vi "Read_Array_of_Products_from_File.vi"(11 "Path":path) -> (3 "Array":T1[](array[typedef]))   [LabVIEW 2020]
doc: "This VI reads <b>array of #typedef Products </b> saved in text file stored in location gived by a <b>path</b>. In file every element of cluster is seperated by comma."
uses:
  #typedef_Product.ctl
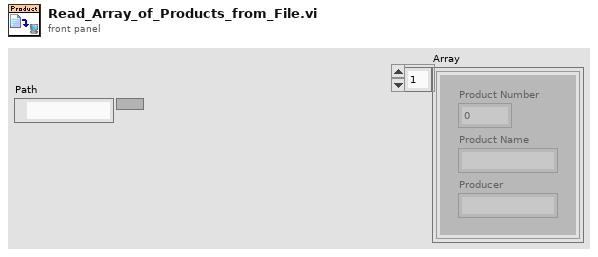
[diagram p1: front panel]
types:
  T1 = typedef "#typedef_Product.ctl" = cluster{"Product Number":i32, "Product Name":string, "Producer":string}
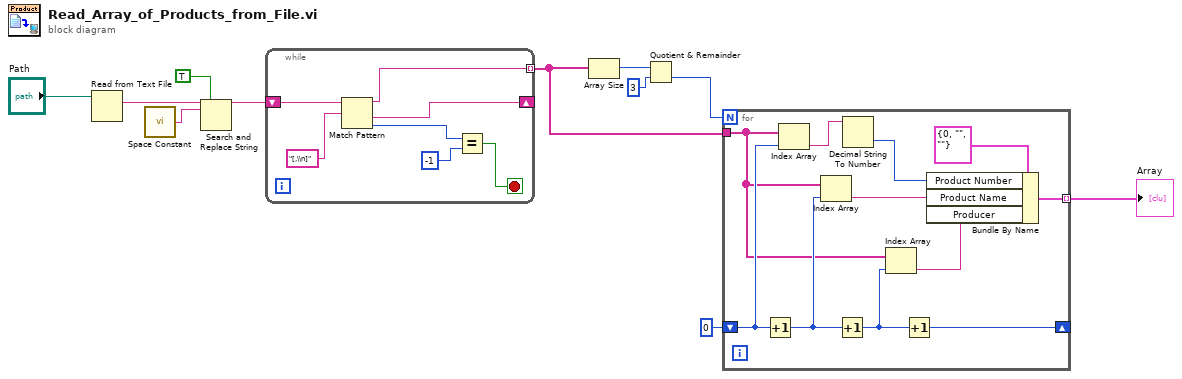
[diagram p0: block diagram]
diagram:
  n1 = Read from Text File(file (use dialog)="Path") -> (text=w8:string)  [unwired: 3 in, 3 out]
  n2 = call <vilib>:"Space Constant.vi"() -> ("String"=w9:string)
  n3 = Search and Replace String(replace all?=TRUE ("replace all? (F)"), input string=w8, search string=w9) -> (result string=w10:string)  [unwired: 5 in, 3 out]
  n4 = while {
    shift-right: [w14] -> _
    shift-left: w10 -> [w13]
    tunnel: [w12] -> w7 mode=indexing
    stop <- w15 stop-if-true
    n5 = Match Pattern(string=w13, regular expression="[,\\n]") -> (before substring=w12:string, after substring=w14:string, offset past match=w17:i32)  [unwired: 1 in, 1 out]
    n6 = Equal?(x=w17, y=-1) -> (x = y?=w15:bool)
  }
  n7 = Array Size(array=w7) -> (size(s)=w3:i32)
  n8 = Quotient & Remainder(x=w3, y=3) -> (floor(x/y)=w5:i32)  [unwired: 1 out]
  n9 = for {
    N: w5 -> [_]
    tunnel: w7 -> [w26]
    shift-right: [w24] -> _
    shift-left: 0 -> [w29]
    tunnel: [w21] -> w1 mode=indexing
    n10 = Increment(x=w29) -> (x+1=w27:i32)
    n11 = Index Array(array=w26, index=w29) -> (element=w28:string)
    n12 = Index Array(array=w26, index=w27) -> (element=w23:string)
    n13 = Increment(x=w27) -> (x+1=w25:i32)
    n14 = Decimal String To Number(string=w28) -> (number=w20:i32)  [unwired: 2 in, 1 out]
    n15 = Index Array(array=w26, index=w25) -> (element=w22:string)
    n16 = Increment(x=w25) -> (x+1=w24:i32)
    n17 = Bundle By Name(cluster=T1 {"Product Number"=0, "Product Name"="", "Producer"=""} ("Product"), "Product Number"=w20, "Product Name"=w23, "Producer"=w22) -> (w21:T1)
  }
  "Array" <- w1
